vi "串口调试.vi"(6 "stop bits (10: 1 bit)":u16(ring)=10 caption="停止位（10: 1位）" items=["1.0"=10, "1.5"=15, "2.0"=20], 7 "写入缓冲区":string, 8 "parity (0:none)":enum16{"None", "Odd", "Even", "Mark", "Space"}(ring) caption="奇偶（0:无）", 9 "data bits (8)":u16=8 caption="数据比特(8)" min=5 max=8 step=1, 10 "baud rate (9600)":u32=9600 caption="波特率(9600)", 11 "VISA resource name":refnum<visa-resource-name> caption="VISA资源名称") -> (1 "OK":bool, 3 "读取缓冲区":string)   [LabVIEW 2015]
uses:
  <vilib>/Instr/_visa.llb/VISA Configure Serial Port (Instr).vi
panel:
  out "error?":bool caption="错误？"
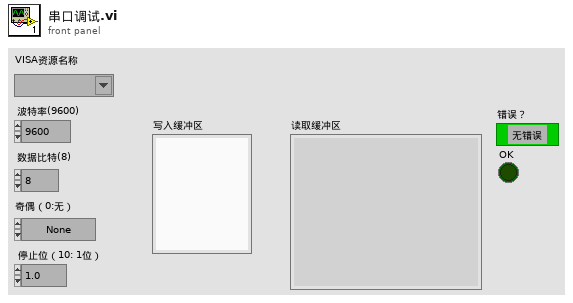
[diagram p1: front panel]
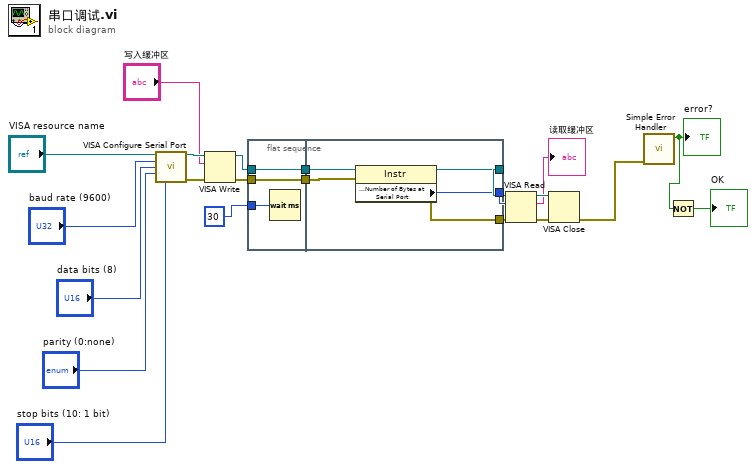
[diagram p0: block diagram]
diagram:
  n1 = call-poly "VISA Configure Serial Port"("VISA resource name"="VISA resource name", "baud rate (9600)"="baud rate (9600)", "data bits (8)"="data bits (8)", "parity (0:none)"="parity (0:none)", "stop bits (10: 1 bit)"="stop bits (10: 1 bit)") -> ("VISA resource name out"=w17:refnum<visa-resource-name>, "error out"=w14:errorcluster)  [unwired: 9 in]
  n2 = VISA Write(VISA resource name=w17, write buffer="写入缓冲区", error in (no error)=w14) -> (VISA resource name out=w10:refnum<visa-resource-name>, error out=w8:errorcluster)  [unwired: 1 out]
  n3 = flat-sequence {
    tunnel: w8 -> [w24]
    tunnel: w10 -> [w25]
    tunnel: [w25] -> w6
    tunnel: [w24] -> w5
    tunnel: u32 30 ("等待时间（毫秒）") -> [w23]
    tunnel: [w30] -> w22
    tunnel: [w28] -> w9
    tunnel: [w26] -> w7
    tunnel: w6 -> [w29]
    tunnel: w5 -> [w27]
    frame #0 {
      n4 = Wait (ms)(milliseconds to wait=w23) -> ()  [unwired: 1 out]
    }
    frame #1 {
      n5 = property class="Instr"(reference=w29, error in=w27) -> (reference out=w28:refnum<visa-resource-name>, error out=w26:errorcluster, "Serial Settings:Number of Bytes at Serial Port"=w30:u32)
    }
  }
  n6 = VISA Read(VISA resource name=w9, byte count=w22, error in (no error)=w7) -> (VISA resource name out=w16:refnum<visa-resource-name>, read buffer=→"读取缓冲区":string, error out=w15:errorcluster)  [unwired: 1 out]
  n7 = VISA Close(VISA resource name=w16, error in (no error)=w15) -> (error out=w1:errorcluster)
  n8 = call <vilib>:"Simple Error Handler.vi"("error in (no error)"=w1) -> ("error?"=w3:bool)  [unwired: 4 in, 4 out]
  "error?" <- w3
  n9 = Not(x=w3) -> (.not. x?=→"OK":bool)
